vi "ShowHideSplit.vi"(1 "Splitter in":refnum<vi>, 2 "Show Split":bool) -> ()   [LabVIEW 2020]
uses:
  5dab802b-0bd9-4eee-8fe3-d4457a3e371f.vi
panel:
  out "error out":errorcluster
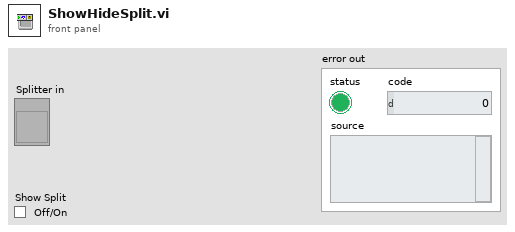
[diagram p1: front panel]
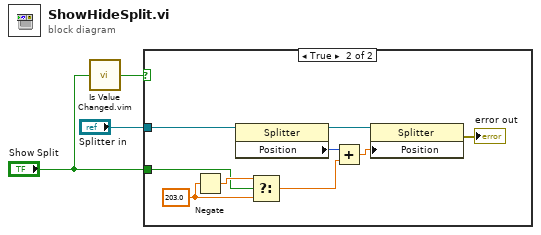
[diagram p0: block diagram]
diagram:
  n1 = call "Is Value Changed.vim"("value"="Show Split") -> ("changed or first call?"=w1:bool)
  n2 = case shown="True" w1 {
    tunnel: "Splitter in" -> [_ w6]
    tunnel: "Show Split" -> [_ w5]
    frame False {
    }
    frame True {
      w11 = 203.0
      n3 = Negate(x=w11) -> (-x=w12:dbl)
      n4 = property class="Splitter"(reference=w6) -> (reference out=w7:refnum<vi>, "Position"=w8:i32)  [unwired: 1 in, 1 out]
      n5 = Select(t=w12, s=w5, f=w11) -> (s? t:f=w10:dbl)
      n6 = Add(x=w8, y=w10) -> (x+y=w9:dbl)
      n7 = property class="Splitter"(reference=w7, "Position"=w9) -> (error out=→"error out":errorcluster)  [unwired: 1 in, 1 out]
    }
  }
